vi "Legacy Serial Comms.vi"(8 "error in (no error)":errorcluster, 11 "VISA Refnum in":refnum<visa-resource-name>) -> (0 "error out":errorcluster, 2 "Numeric":dbl, 3 "Numeric 2":dbl)   [LabVIEW 2019]
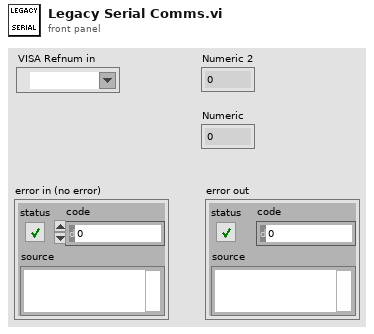
[diagram p1: front panel]
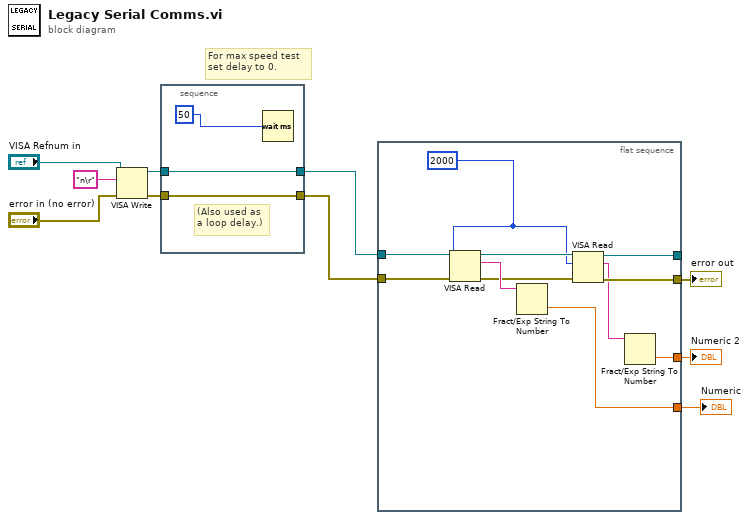
[diagram p0: block diagram]
diagram:
  # "For max speed test \nset delay to 0."
  n1 = VISA Write(VISA resource name="VISA Refnum in", write buffer="n\r" ("String to Write"), error in (no error)="error in (no error)") -> (VISA resource name out=w4:refnum<visa-resource-name>, error out=w2:errorcluster)  [unwired: 1 out]
  n2 = stacked-sequence {
    tunnel: w2 -> [w13]
    tunnel: [w13] -> w3
    tunnel: w4 -> [w12]
    tunnel: [w12] -> w5
    frame #0 {
      # "(Also used as\na loop delay.)"
      n3 = Wait (ms)(milliseconds to wait=u32 50 ("t")) -> ()  [unwired: 1 out]
    }
  }
  n4 = flat-sequence {
    tunnel: w3 -> [w24]
    tunnel: w5 -> [w23]
    tunnel: [w22] -> _
    tunnel: [w21] -> w1
    tunnel: [w15] -> w10
    tunnel: [w14] -> w9
    frame #0 {
      w17 = u32 2000 ("byte count")
      n5 = VISA Read(VISA resource name=w23, byte count=w17, error in (no error)=w24) -> (VISA resource name out=w19:refnum<visa-resource-name>, read buffer=w20:string, error out=w18:errorcluster)  [unwired: 1 out]
      n6 = Fract/Exp String To Number(string=w20) -> (number=w15:dbl)  [unwired: 3 in, 1 out]
      n7 = VISA Read(VISA resource name=w19, byte count=w17, error in (no error)=w18) -> (VISA resource name out=w22:refnum<visa-resource-name>, read buffer=w16:string, error out=w21:errorcluster)  [unwired: 1 out]
      n8 = Fract/Exp String To Number(string=w16) -> (number=w14:dbl)  [unwired: 3 in, 1 out]
    }
  }
  "Numeric" <- w10
  "Numeric 2" <- w9
  "error out" <- w1
